vi "LC Load File.vi"(8 "error in (no error)":errorcluster caption="错误输入（无错误）", 9 "Parent Tag":string, 10 "VI Path":refnum<vi>, 11 "selected path":path) -> (0 "error out":errorcluster caption="错误输出")   [LabVIEW 2020]
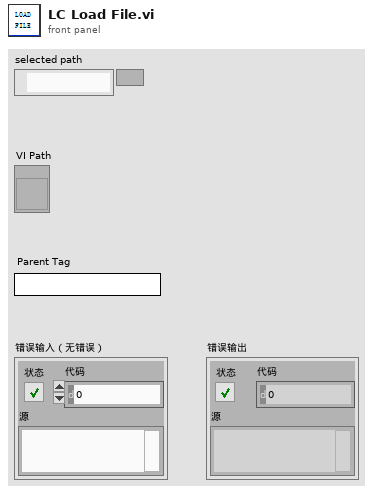
[diagram p1: front panel]
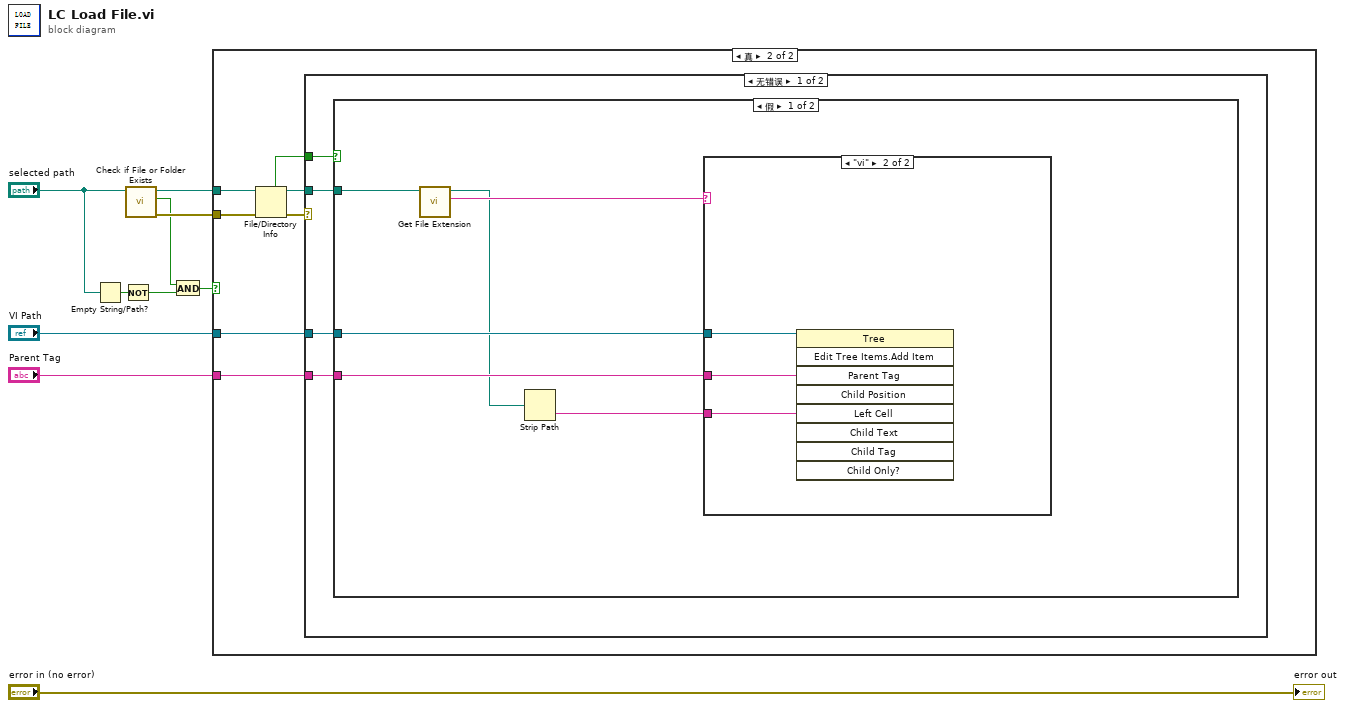
[diagram p0: block diagram]
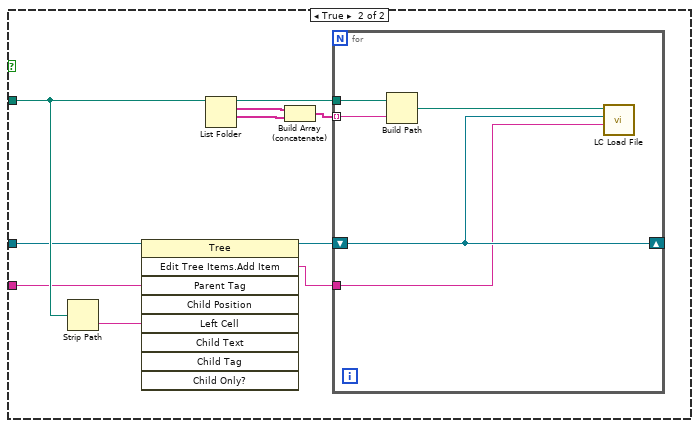
[diagram p4: hidden frame]
diagram:
  n1 = Empty String/Path?(string/path="selected path") -> (empty?=w4:bool)
  n2 = Not(x=w4) -> (.not. x?=w2:bool)
  n3 = call <vilib>:"Check if File or Folder Exists.vi"("path"="selected path") -> ("error out"=w6:errorcluster, "file or folder exists?"=w3:bool, "dup path"=w7:path)  [unwired: 8 in]
  n4 = And(x=w3, y=w2) -> (x .and. y?=w1:bool)
  n5 = case shown="真" w1 {
    tunnel: "Parent Tag" -> [_ w14]
    tunnel: "VI Path" -> [_ w13]
    tunnel: w7 -> [_ w12]
    tunnel: w6 -> [_ w11]
    frame False {
    }
    frame True {
      n6 = File/Directory Info(path=w12, error in=w11) -> (path out=w16:path, directory=w17:bool, error out=w15:errorcluster)  [unwired: 4 out]
      n7 = case shown="无错误" w15 {
        tunnel: w17 -> [w21 _]
        tunnel: w16 -> [w20 _]
        tunnel: w14 -> [w19 _]
        tunnel: w13 -> [w18 _]
        frame No Error {
          n8 = case shown="假" w21 {
            tunnel: w20 -> [w27 w39]
            tunnel: w19 -> [w25 w36]
            tunnel: w18 -> [w26 w38]
            frame False {
              n9 = call <vilib>:"Get File Extension.vi"("file"=w27) -> ("lowercase file extension"=w24:string, "dup file"=w23:path)  [unwired: 6 in, 3 out]
              n10 = Strip Path(path=w23) -> (name=w22:string)  [unwired: 1 out]
              n11 = case shown="\"vi\"" w24 {
                tunnel: w26 -> [_ w30]
                tunnel: w25 -> [_ w29]
                tunnel: w22 -> [_ w28]
                frame "eee", Default {
                }
                frame "vi" {
                  n12 = invoke class="Tree" method="Edit Tree Items.Add Item"(reference=w30, "Parent Tag"=w29, "Left Cell"=w28) -> ()  [unwired: 6 in, 9 out]
                }
              }
            }
            frame True {
              n13 = Strip Path(path=w39) -> (name=w35:string)  [unwired: 1 out]
              n14 = invoke class="Tree" method="Edit Tree Items.Add Item"(reference=w38, "Parent Tag"=w36, "Left Cell"=w35) -> (reference out=w37:refnum<vi>, "Edit Tree Items:Add Item"=w34:string)  [unwired: 6 in, 7 out]
              n15 = List Folder(path=w39) -> (path out=w40:path, filenames=w33:string[], folder names=w32:string[])  [unwired: 3 in, 1 out]
              n16 = Build Array (concatenate)(w33, w32) -> (w31:string[])
              n17 = for {
                tunnel: w40 -> [w45]
                tunnel: w31 -> [w44] mode=indexing
                tunnel: w34 -> [w41]
                shift-right: [w43] -> _
                shift-left: w37 -> [w43]
                n18 = Build Path(base path=w45, name or relative path=w44) -> (appended path=w42:path)
                n19 = call "LC Load File.vi"("Parent Tag"=w41, "VI Path"=w43, "selected path"=w42) -> ()  [unwired: 8 in, 1 out]
              }
            }
          }
        }
        frame Error {
        }
      }
    }
  }
  "error out" <- "error in (no error)"
